vi "_FPGA Read Key.vi"(5 "error in (no error)":errorcluster, 6 "CurStartupMode (0)":u8, 7 "ForStart (F)":bool) -> (0 "error out":errorcluster, 1 "Key Pressed":bool, 3 "Key Pressed 2":bool)   [LabVIEW 2015]
uses:
  Type/_RT LED Num.ctl
  _RT Global.vi
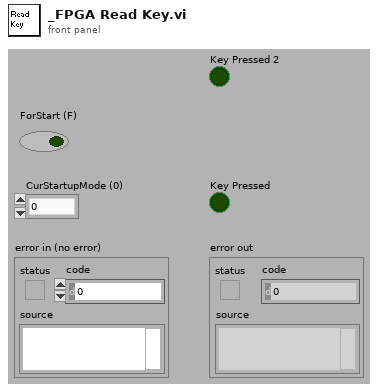
[diagram p1: front panel]
types:
  T1 = typedef "_RT LED Num.ctl" = enum8{"ReadKey", "ClearKeyBuffer", "ClearLCD", "BacklightOn"}
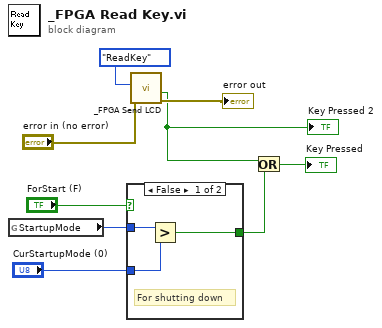
[diagram p0: block diagram]
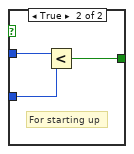
[diagram p2: hidden frame]
diagram:
  n1 = global read "_RT Global.vi" "StartupMode"() -> (w4:u8)
  n2 = case shown="False" "ForStart (F)" {
    tunnel: w4 -> [w12 w15]
    tunnel: "CurStartupMode (0)" -> [w11 w14]
    tunnel: [w10 w13] -> w2
    frame False {
      # "For shutting down"
      n3 = Greater?(x=w12, y=w11) -> (0:w10:bool)
    }
    frame True {
      # "For starting up"
      n4 = Less?(x=w15, y=w14) -> (x < y?=w13:bool)
    }
  }
  n5 = call "_FPGA Send LCD.vi"("error in (no error)"="error in (no error)", "Command"=_RT_LED_Num."ReadKey" ("LED#")) -> ("error out"=→"error out":errorcluster, "Key Pressed"=w1:bool)  [unwired: 3 in, 2 out]
  "Key Pressed 2" <- w1
  n6 = Or(x=w1, y=w2) -> (x .or. y?=→"Key Pressed":bool)
